vi "Client.vi"() -> ()   [LabVIEW 2017]
panel:
  in  "stop 3":bool
  out "Waveform Chart 2":cluster{dbl}(graph)
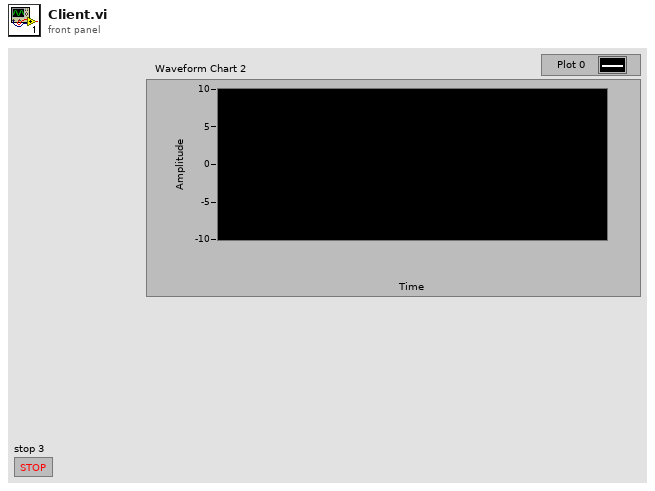
[diagram p1: front panel]
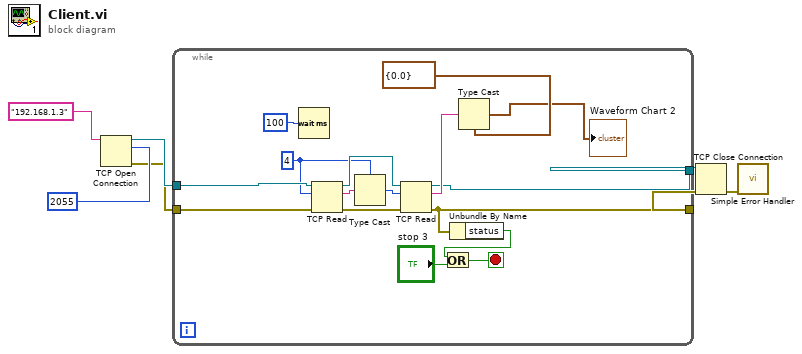
[diagram p0: block diagram]
diagram:
  n1 = TCP Open Connection(address="192.168.1.3", remote port or service name=u16 2055) -> (connection ID=w6:refnum<k5>, error out=w4:errorcluster)  [unwired: 3 in]
  n2 = while {
    tunnel: w6 -> [w23]
    tunnel: w4 -> [w21]
    tunnel: [w14] -> w3
    tunnel: [w10] -> w2
    stop <- w12 stop-if-true
    w17 = 4 ("bytes to read")
    n3 = Wait (ms)(milliseconds to wait=u32 100) -> ()  [unwired: 1 out]
    n4 = TCP Read(connection ID=w23, bytes to read=w17, error in (no error)=w21) -> (connection ID out=w19:refnum<k5>, data out=w18:string, error out=w20:errorcluster)  [unwired: 2 in]
    n5 = Type Cast(type=w17, x=w18) -> (*(type *) &x=w16:i32)
    n6 = TCP Read(connection ID=w19, bytes to read=w16, error in (no error)=w20) -> (connection ID out=w14:refnum<k5>, data out=w15:string, error out=w10:errorcluster)  [unwired: 2 in]
    n7 = Unbundle By Name(w10) -> ("status"=w9:bool)
    n8 = Or(x=w9, y="stop 3") -> (x .or. y?=w12:bool)
    n9 = Type Cast(type=cluster{dbl} {0.0}, x=w15) -> (*(type *) &x=→"Waveform Chart 2":cluster{dbl})
  }
  n10 = TCP Close Connection(connection ID=w3, error in (no error)=w2) -> (error out=w1:errorcluster)  [unwired: 1 in, 1 out]
  n11 = call <vilib>:"Simple Error Handler.vi"("error in (no error)"=w1) -> ()  [unwired: 4 in, 5 out]
